vi "ReceiveInstructionData.vi"(6 "Timeout ms":i32=1, 7 "UDP Input":T2) -> (0 "Error Out":errorcluster, 1 "MotorInstuction Output":T1, 2 "Did Receive":bool, 3 "UDP Output":T2)   [LabVIEW 2019]
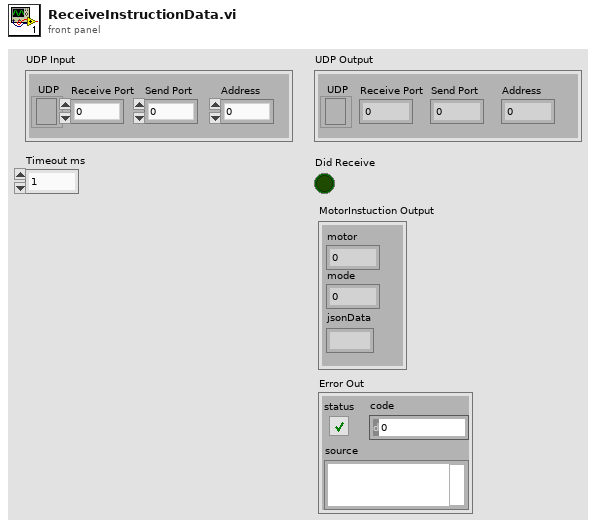
[diagram p1: front panel]
types:
  T1 = cluster{"motor":i8, "mode":i8, "jsonData":string}
  T2 = cluster{"UDP":refnum<k16>, "Receive Port":i32, "Send Port":i32, "Address":i64}
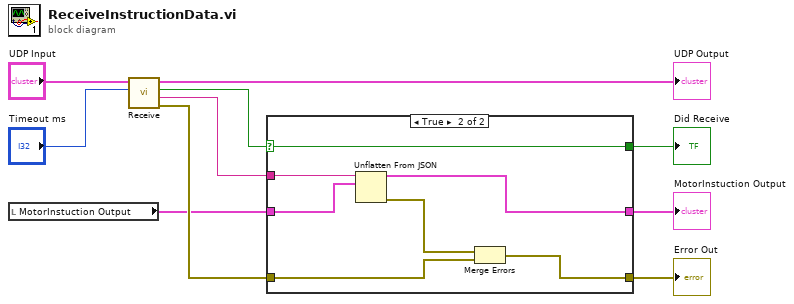
[diagram p0: block diagram]
diagram:
  n1 = local read "MotorInstuction Output"() -> (w1:T1)
  n2 = call "Receive.vi"("Timeout ms"="Timeout ms", "UDP Input"="UDP Input") -> ("Error Out"=w7:errorcluster, "Received Data"=w3:string, "Did Receive"=w5:bool, "UDP Output"=→"UDP Output":T2)  [unwired: 2 in]
  n3 = case shown="True" w5 {
    selector: w5 -> [w11 w15]
    tunnel: w1 -> [w13 w20]
    tunnel: [w12 w18] -> w6
    tunnel: [w13 w19] -> w2
    tunnel: w7 -> [w12 w16]
    tunnel: [w11 w15] -> w4
    tunnel: w3 -> [_ w14]
    frame False {
    }
    frame True {
      n4 = Unflatten From JSON(JSON string=w14, type and defaults=w20) -> (value=w19:T1, error out=w17:errorcluster)  [unwired: 5 in]
      n5 = Merge Errors(w17, w16) -> (w18:errorcluster)
    }
  }
  "Error Out" <- w6
  "Did Receive" <- w4
  "MotorInstuction Output" <- w2
